vi "TX ADU.vi"(8 "error in (no error)":errorcluster, 9 "PDU_req in":T1={"Function Code"=1, "Data"=[], "RTU_DataBytes"=0}, 10 "VISA resource in":refnum<visa-resource-name>, 11 "MB_ADU in":refnum<class "MB_ADU_RTU.lvclass">) -> (0 "error out":errorcluster, 1 "PDU_req out":T1={"Function Code"=1, "Data"=[], "RTU_DataBytes"=0}, 2 "VISA resource out":refnum<visa-resource-name>, 3 "MB_ADU out":refnum<class "MB_ADU_RTU.lvclass">)   [LabVIEW 2012, in "MB Master.lvlib" / "MB_ADU_RTU.lvclass"]
doc: "Defines the transmit procedure for a Modbus RTU ADU. The PDU to be transmitted should be written to PDU_req prior to calling this VI."
uses:
  MB_ADU_RTU.lvclass
  MB_PDU/MB_PDU_Cluster.ctl
  MB_ADU/MB_ADU.lvclass/MB_ADU.ctl
  MB_ADU_RTU.lvclass/MB_ADU_RTU.ctl
  MB_ADU/Read Slave ID.vi
  MB_ADU/Write TX Data.vi
  MB_ADU/Write TX Timestamp.vi
  MB Master.lvlib
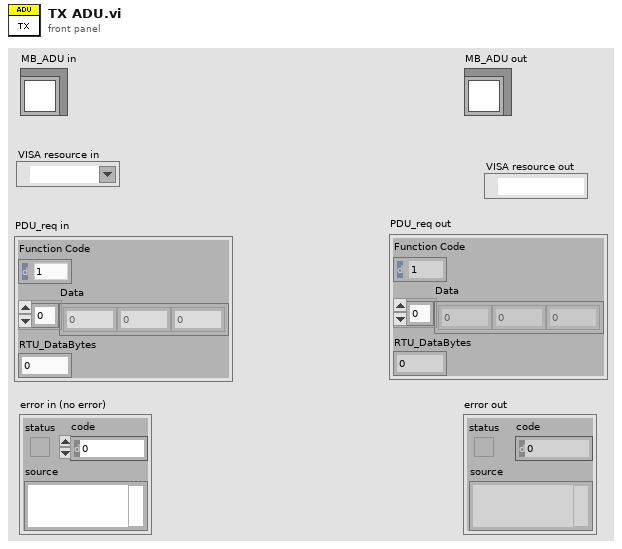
[diagram p1: front panel]
types:
  T1 = typedef "MB Master.lvlib/MB_PDU_Cluster.ctl" = cluster{"Function Code":u8, "Data":u8[], "RTU_DataBytes":i32}
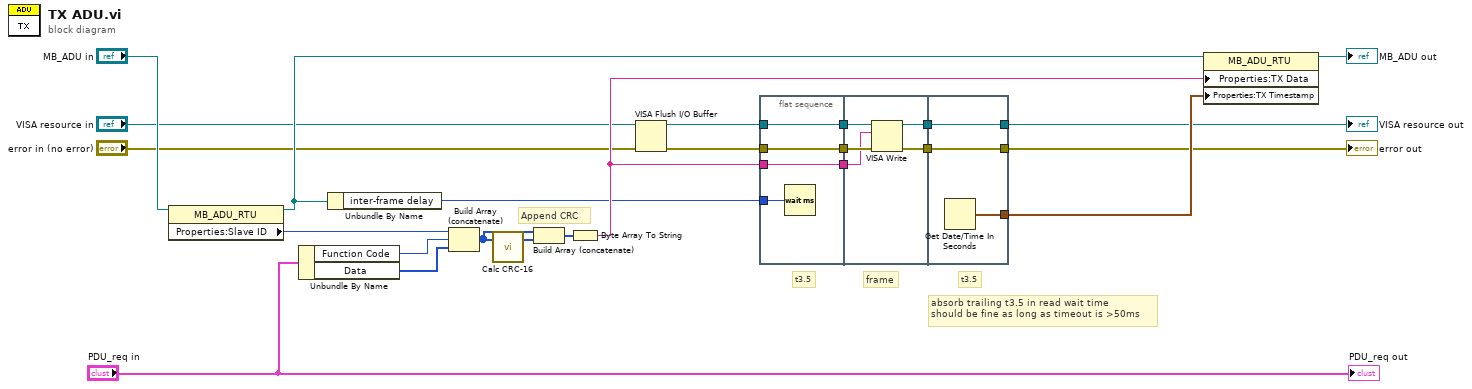
[diagram p0: block diagram]
diagram:
  # "absorb trailing t3.5 in read wait time\nshould be fine as long as timeout is >50ms"
  # "frame"
  # "t3.5"
  # "t3.5"
  # "Append CRC"
  n1 = property class="MB_ADU_RTU"(reference="MB_ADU in") -> (reference out=w9:refnum<class "MB_ADU_RTU.lvclass">, "Properties:Slave ID"=w23:u8)  [unwired: 1 in, 1 out]
  n2 = Unbundle By Name("PDU_req in") -> ("Function Code"=w3:u8, "Data"=w2:u8[])
  n3 = Unbundle By Name(w9) -> ("inter-frame delay"=w8:u32)
  n4 = Build Array (concatenate)(w23, w3, w2) -> (w21:u8[])
  n5 = call "Calc CRC-16.vi"("Frame in"=w21) -> ("CRC-16"=w22:u8[])  [unwired: 2 in]
  n6 = Build Array (concatenate)(w21, w22) -> (w20:u8[])
  n7 = Byte Array To String(unsigned byte array=w20) -> (string=w15:string)
  n8 = VISA Flush I/O Buffer(VISA resource name="VISA resource in", error in (no error)="error in (no error)") -> (VISA resource name out=w7:refnum<visa-resource-name>, error out=w6:errorcluster)  [unwired: 1 in]
  n9 = flat-sequence {
    tunnel: [w28] -> w12
    tunnel: [w27] -> w11
    tunnel: [w26] -> w10
    tunnel: w7 -> [w28]
    tunnel: w6 -> [w27]
    tunnel: w15 -> [w26]
    tunnel: w8 -> [w25]
    tunnel: [w30] -> w18
    tunnel: [w29] -> w17
    tunnel: w10 -> [w31]
    tunnel: w11 -> [w32]
    tunnel: w12 -> [w33]
    tunnel: [w35] -> w13
    tunnel: [w36] -> w14
    tunnel: [w34] -> w16
    tunnel: w17 -> [w35]
    tunnel: w18 -> [w36]
    frame #0 {
      n10 = Wait (ms)(milliseconds to wait=w25) -> ()  [unwired: 1 out]
    }
    frame #1 {
      n11 = VISA Write(VISA resource name=w33, write buffer=w31, error in (no error)=w32) -> (VISA resource name out=w30:refnum<visa-resource-name>, error out=w29:errorcluster)  [unwired: 1 out]
    }
    frame #2 {
      n12 = Get Date/Time In Seconds() -> (seconds since 1Jan1904=w34:timestamp)
    }
  }
  n13 = property class="MB_ADU_RTU"(reference=w9, "Properties:TX Data"=w15, "Properties:TX Timestamp"=w16) -> (reference out=→"MB_ADU out":refnum<class "MB_ADU_RTU.lvclass">)  [unwired: 1 in, 1 out]
  "error out" <- w13
  "VISA resource out" <- w14
  "PDU_req out" <- "PDU_req in"
